vi "Active Actor Monitor.vi"(7 "Write? (f)":bool, 10 "Monitor Type in":refnum<class "Actor Monitor.lvclass">) -> (2 "Monitor Type out":refnum<class "Actor Monitor.lvclass">)   [LabVIEW 2017, in "MGI-Monitored Actor Core.lvlib"]
doc: "Functional global that stores the type of actor monitor to use\n\nCopyright: MGI 2016\nAuthor: Derek Trepanier"
uses:
  MGI-Monitored Actor Core.lvlib
  Actor Monitor/Actor Monitor/Actor Monitor.lvclass
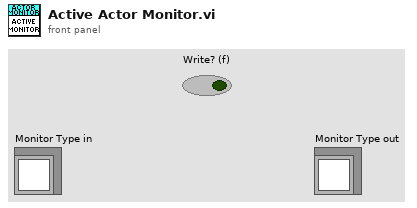
[diagram p1: front panel]
types:
  T1 = enum32{"invalid app kind", "Development System", "Run Time System", "Student Edition", "Embedded LabVIEW", "Evaluation", "Custom"}
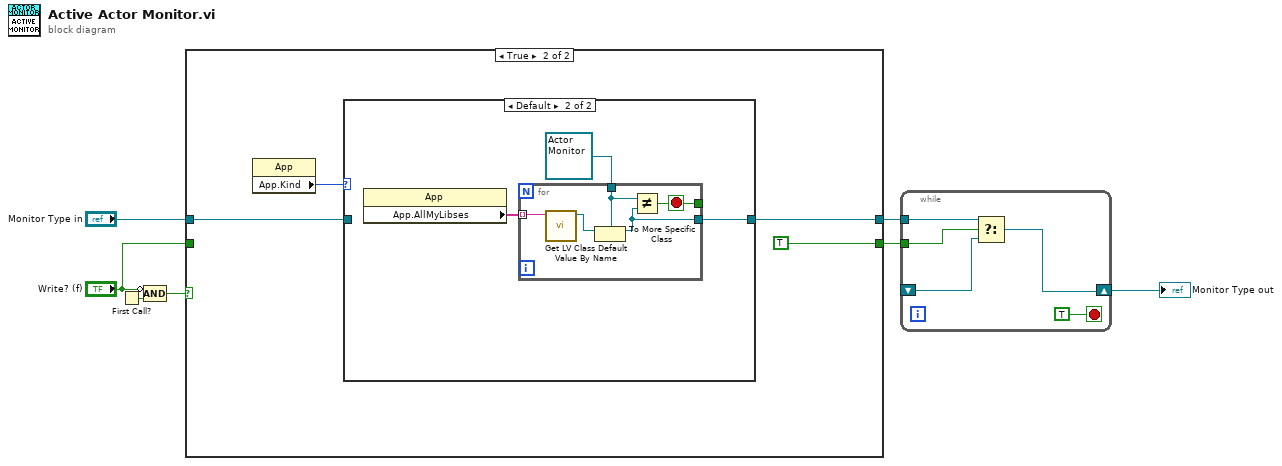
[diagram p0: block diagram]
diagram:
  n1 = First Call?() -> (First Call?: T/F=w6:bool)
  n2 = Compound Arithmetic op=AND(invert "Write? (f)", w6) -> (w5:bool)
  n3 = case shown="True" w5 {
    tunnel: [w9 w13] -> w4
    tunnel: "Monitor Type in" -> [w9 w10]
    tunnel: [w8 TRUE] -> w2
    tunnel: "Write? (f)" -> [w8 _]
    frame False {
    }
    frame True {
      n4 = property class="App"() -> ("App.Kind"=w11:T1)  [unwired: 2 in, 2 out]
      n5 = case shown="Default" w11 {
        tunnel: [w14 w17] -> w13
        tunnel: w10 -> [w14 _]
        frame "Run Time System" {
        }
        frame Default {
          n6 = property class="App"() -> ("App.AllMyLibses"=w16:string[])  [unwired: 2 in, 2 out]
          n7 = for {
            tunnel: w16 -> [w22] mode=indexing
            tunnel: refnum<class "Actor Monitor.lvclass"> refnum ("Monitored Actor.lvlib:Actor Monitor.lvclass") -> [w19]
            tunnel: [w20] -> w17
            tunnel: [w18] -> _
            stop <- w18 stop-if-true
            n8 = call <vilib>:"Get LV Class Default Value By Name.vi"("class name"=w22) -> ("object"=w21:refnum<class>)  [unwired: 9 in, 1 out]
            n9 = To More Specific Class(target class=w19, reference=w21) -> (specific class reference=w20:refnum<class "Actor Monitor.lvclass">)  [unwired: 1 in, 1 out]
            n10 = Not Equal?(x=w19, y=w20) -> (x != y?=w18:bool)
          }
        }
      }
    }
  }
  n11 = while {
    tunnel: w4 -> [w26]
    tunnel: w2 -> [w25]
    shift-right: [w24] -> w7
    shift-left: _ -> [w23]
    stop <- TRUE stop-if-true
    n12 = Select(t=w26, s=w25, f=w23) -> (s? t:f=w24:refnum<class "Actor Monitor.lvclass">)
  }
  "Monitor Type out" <- w7
